vi "Remove (EventToken).vi"(8 "error in (no error)":errorcluster, 9 "EventToken":refnum<class "EventToken.lvclass">, 11 "EventBag in":refnum<class "EventBag.lvclass">) -> (0 "error out":errorcluster, 3 "EventBag out":refnum<class "EventBag.lvclass">)   [LabVIEW 2009, in "EventManagerLibrary.lvlib" / "EventBag.lvclass"]
uses:
  EventBag.lvclass
  EventToken/EventToken.lvclass
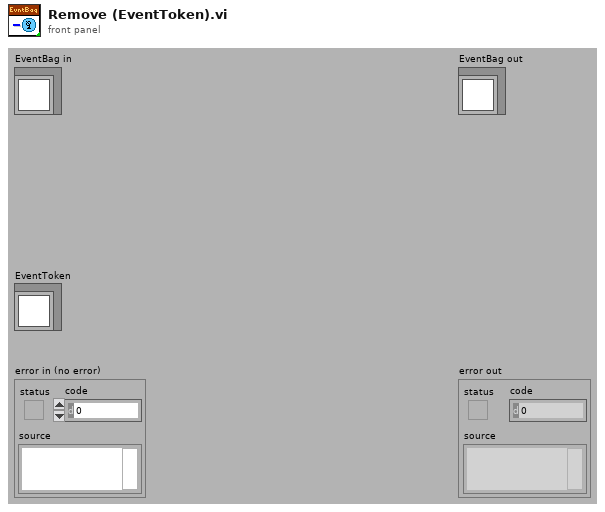
[diagram p1: front panel]
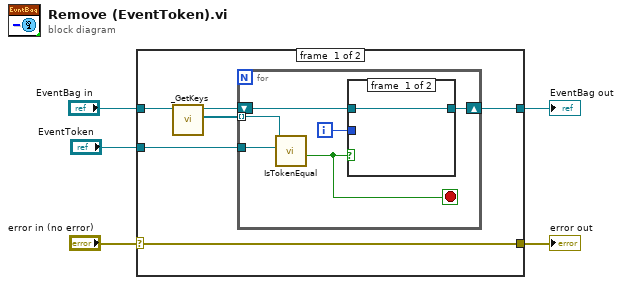
[diagram p0: block diagram]
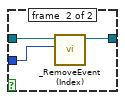
[diagram p2: hidden frame]
diagram:
  n1 = case shown="No Error" "error in (no error)" {
    selector: "error in (no error)" -> [w7 w23]
    tunnel: [w7 w23] -> w2
    tunnel: [w8 w22] -> w4
    tunnel: "EventBag in" -> [w11 w22]
    tunnel: "EventToken" -> [w6 _]
    frame #0 {
      n2 = call "_GetKeys.vi"("EventBag in"=w11) -> ("Keys"=w10:refnum<class "EventToken.lvclass">[], "EventBag out"=w9:refnum<class "EventBag.lvclass">)  [unwired: 8 in, 1 out]
      n3 = for {
        tunnel: w10 -> [w13] mode=indexing
        shift-right: [w16] -> w8
        shift-left: w9 -> [w17]
        tunnel: w6 -> [w12]
        i -> [w15]
        stop <- w14 stop-if-true
        n4 = call-dynamic "IsTokenEqual.vi"("EventToken"=w12, "EventToken in"=w13) -> ("Is Equal?"=w14:bool)  [unwired: 6 in, 3 out]
        n5 = case shown="True" w14 {
          tunnel: w17 -> [w18 w21]
          tunnel: [w18 w19] -> w16
          tunnel: w15 -> [_ w20]
          frame #0 {
          }
          frame #1 {
            n6 = call "_RemoveEvent (Index).vi"("Index"=w20, "EventBag in"=w21) -> ("EventBag out"=w19:refnum<class "EventBag.lvclass">)  [unwired: 8 in, 1 out]
          }
        }
      }
    }
    frame #1 {
    }
  }
  "error out" <- w2
  "EventBag out" <- w4
